vi "Write String.vi"(8 "error in (no error)":errorcluster, 10 "String":string, 11 "Event in":refnum<class "Event String.lvclass">) -> (0 "error out":errorcluster, 3 "Event out":refnum<class "Event String.lvclass">)   [LabVIEW 2017, in "Event Actors.lvlib" / "Event String.lvclass"]
uses:
  Event String.lvclass
  Event String.lvclass/Event String.ctl
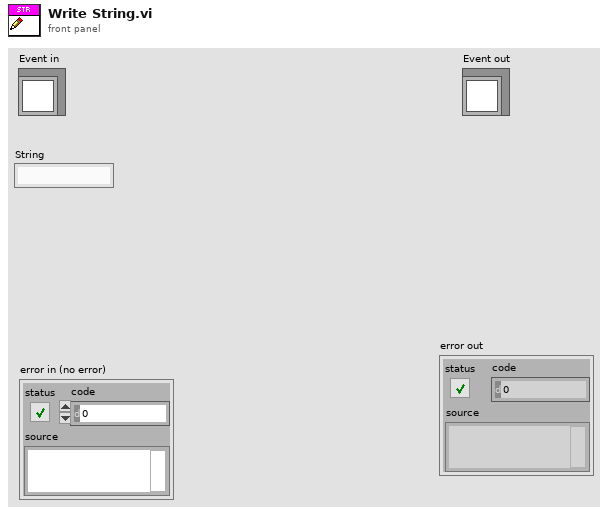
[diagram p1: front panel]
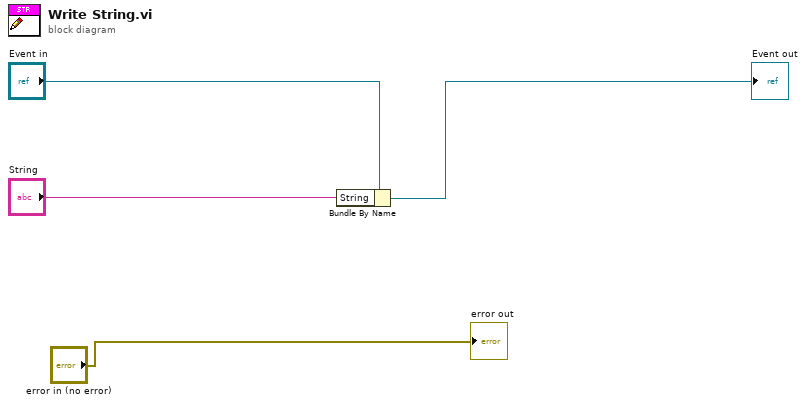
[diagram p0: block diagram]
diagram:
  n1 = Bundle By Name(cluster="Event in", "String"="String") -> (→"Event out":refnum<class "Event String.lvclass">)
  "error out" <- "error in (no error)"
